vi "Apply (Mono 16 Array).vi"(7 "Scaling Factor (Default 1/256)":dbl=0.00390625, 8 "error in (no error)":errorcluster, 9 "Destination Image in":T1, 10 "Mono 16 Image Data":u16[][](array[numeric]), 11 "CLAHE in":refnum<class "CLAHE.lvclass">) -> (0 "error out":errorcluster, 2 "Destination Image":T1, 3 "CLAHE":refnum<class "CLAHE.lvclass">)   [LabVIEW 2020, in "image.lvlib" / "CLAHE.lvclass"]
uses:
  CLAHE.lvclass
  common/common.lvlib
  common/bin/gartoolkit_32-1.dll
  Greyscale Image.ctl
  image.lvlib
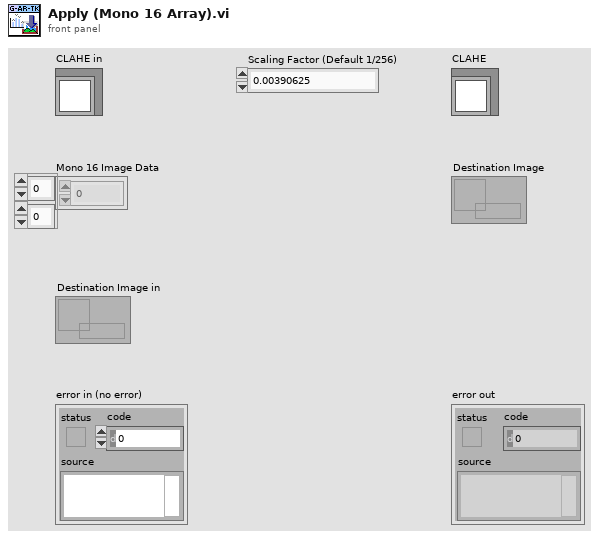
[diagram p1: front panel]
types:
  T1 = typedef "image.lvlib/Greyscale Image.ctl" = refnum<data-value>
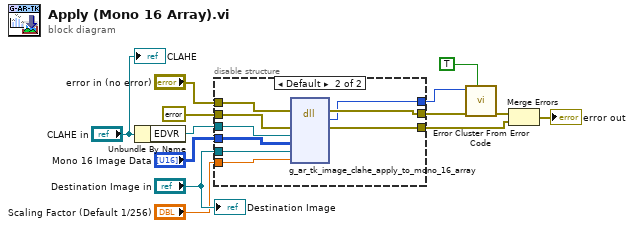
[diagram p0: block diagram]
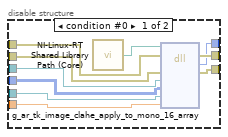
[diagram p2: hidden frame]
diagram:
  n1 = Unbundle By Name("CLAHE in") -> ("EDVR"=w2:refnum<data-value>)
  n2 = disable-structure shown="Default" {
    disable-tunnel: "error in (no error)" -> [w22 w32]
    disable-tunnel: errorcluster {"status"=FALSE, "code"=0, "source"=""} ("error constant") -> [w20 w31]
    disable-tunnel: w2 -> [w19 w27]
    disable-tunnel: [w21 w30] -> w11
    disable-tunnel: [w15 w29] -> w10
    disable-tunnel: [w16 w28] -> w9
    disable-tunnel: "Mono 16 Image Data" -> [w17 w26]
    disable-tunnel: "Destination Image in" -> [w18 w25]
    disable-tunnel: "Scaling Factor (Default 1/256)" -> [w14 w24]
    frame condition #0 {
      n3 = call "NI-Linux-RT Shared Library Path (Core).vi"() -> ("Path"=w23:path)
      n4 = dll-call lib="?" fn="g_ar_tk_image_clahe_apply_to_mono_16_array" ("g_ar_toolkit.*.*:g_ar_tk_image_copy")(path in=w23, error in=w22, "error_cluster"=w20, "EDVR"=w19, "Array"=w17, "Destination"=w18, "Scaling Factor"=w14) -> (error out=w21:errorcluster, "return type"=w15:i32, "error_cluster"=w16:errorcluster)  [unwired: 5 in, 1 out]
    }
    frame condition #1 (active) {
      n5 = dll-call lib="C:/serenial/lib/g-augmented-reality-toolkit/LabVIEW/common/bin/gartoolkit_*-1.*" fn="g_ar_tk_image_clahe_apply_to_mono_16_array" ("g_ar_toolkit.*.*:g_ar_tk_image_copy")(error in=w32, "error_cluster"=w31, "EDVR"=w27, "Array"=w26, "Destination"=w25, "Scaling Factor"=w24) -> (error out=w30:errorcluster, "return type"=w29:i32, "error_cluster"=w28:errorcluster)  [unwired: 6 in, 1 out]
    }
  }
  n6 = call <vilib>:"Error Cluster From Error Code.vi"("show call chain? (False)"=TRUE, "error in (no error)"=w11, "error code (0)"=w10) -> ("error out"=w13:errorcluster)  [unwired: 6 in]
  n7 = Merge Errors(w13, w9) -> (→"error out":errorcluster)
  "CLAHE" <- "CLAHE in"
  "Destination Image" <- "Destination Image in"
